vi "Actor Core.vi"(8 "error in":errorcluster, 11 "MonSys_Client_Actor in":refnum<class "MonSys_Client_Actor.lvclass">) -> (0 "error out":errorcluster, 3 "Actor out":refnum<class "Actor.lvclass">)   [LabVIEW 2018, in "MonSys_Client_Actor.lvlib" / "MonSys_Client_Actor.lvclass"]
doc: "(<B>Filename</B>: Actor Framework.lvlib:Actor.lvclass:Actor Core.vi)\n\nReceives messages to the actor, reacts to them, and initiates any error handling that may shut the actor down.\n\nDescendant classes may override this VI to append parallel tasks for the actor to complete while it handles messages. Overrides use the Call Parent Method node."
uses:
  MonSys_Client_Actor.lvclass
  C:/Program Files (x86)/National Instruments/LabVIEW 2018/vi.lib/ActorFramework/Actor/Actor.lvclass
  <vilib>/ActorFramework/Actor/Actor.lvclass
  _MonSys_LIB/OnlineData.ctl
  _MonSys_LIB/OnlineData_State.ctl
  MonSys_Client_Actor.lvclass/MonSys_Client_Actor.ctl
  <vilib>/ActorFramework/Actor/Actor.lvclass/Actor.ctl
  <vilib>/ActorFramework/Message Enqueuer/Message Enqueuer.lvclass/Message Enqueuer.ctl
  <extravilib>/ChannelInstances/Tag-bool/Read With Abort.vi
  <vilib>/ActorFramework/Message Enqueuer/Init from Existing Queue.vi
  <vilib>/ActorFramework/Message Enqueuer/Enqueue.vi
  <extravilib>/ChannelInstances/Tag-bool/Write With Abort.vi
  <vilib>/ActorFramework/Stop Msg/Stop Msg.lvclass
  C:/Program Files (x86)/National Instruments/LabVIEW 2018/vi.lib/ActorFramework/Message/Message.lvclass
  <extravilib>/ChannelInstances/Tag-bool/Instantiate.vi
  <extravilib>/ChannelInstances/Tag-bool/EndpointRead.vi
  <vilib>/ActorFramework/Message Priority Queue/Priority Enqueue.vi
  <extravilib>/ChannelInstances/Tag-bool/Endpoint.vi
  <vilib>/ActorFramework/Message Enqueuer/Message Enqueuer.lvclass
  <vilib>/httpClient/LabVIEWHTTPClient.lvlib
  <extravilib>/ChannelInstances/Tag-bool.lvlib
  _MonSys_LIB/_MonSys_LIB.lvlib
panel:
  out "selected port":string
  out "selected ip address":string
  in  "request_cycle [ms]":u32=1000
  out "web server connection status":string
  out "value":T1 {"OnlineData_State" items=["Idle", "Manually", "Automatic"]}
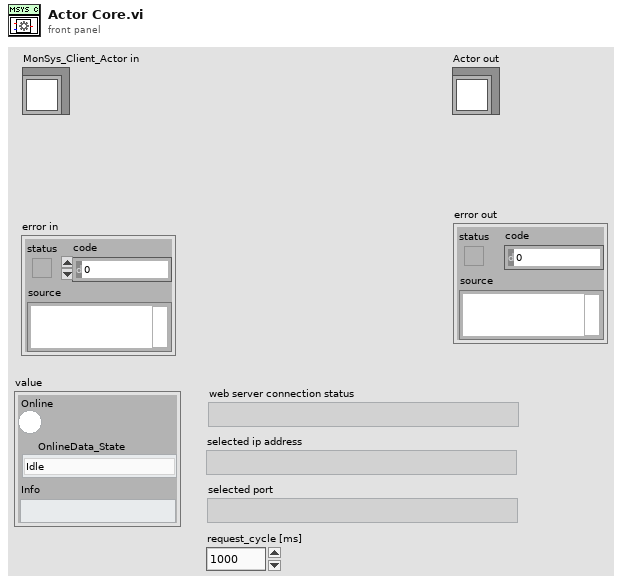
[diagram p1: front panel]
types:
  T1 = typedef "_MonSys_LIB.lvlib/OnlineData.ctl" = cluster{"Online":bool, "Info":string, "OnlineData_State":T2}
  T2 = typedef "_MonSys_LIB.lvlib/OnlineData_State.ctl" = u16
  T3 = enum32{"Invalid", "Standard", "Closed", "Hidden", "Minimized", "Maximized"}
  T4 = typedef "LabVIEWHTTPClient.lvlib/ClientHandle.ctl" = refnum<k1>
  T5 = typedef "Tag-bool.lvlib/))Channel.ctl" = refnum<queue>
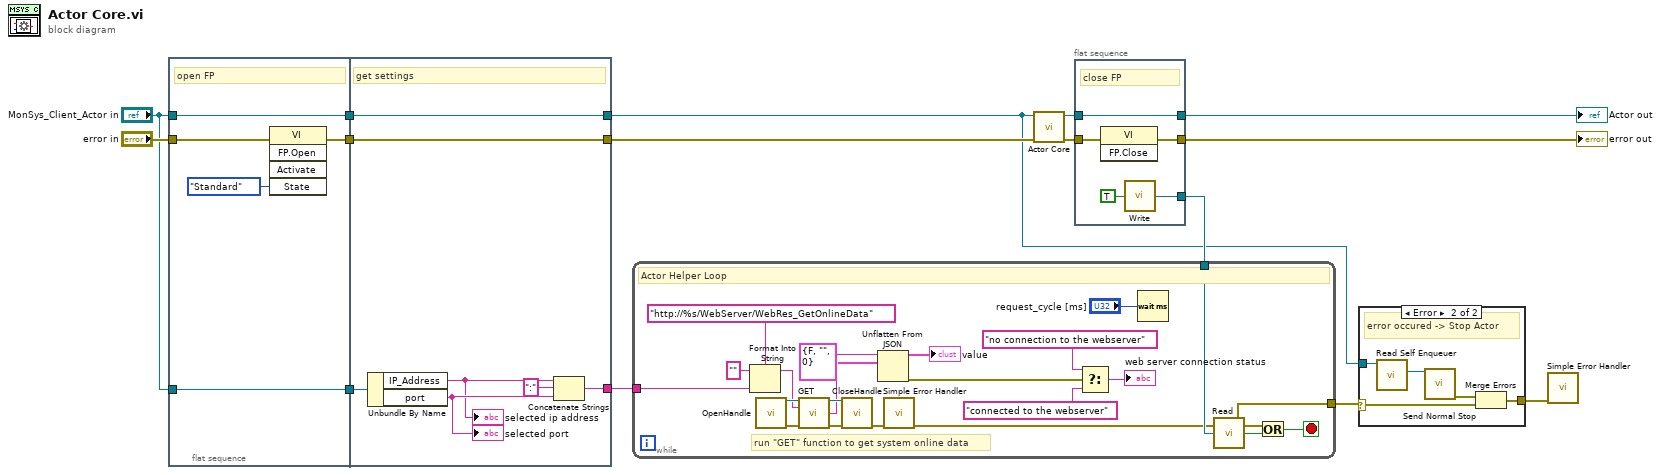
[diagram p0: block diagram]
diagram:
  n1 = flat-sequence {
    tunnel: "MonSys_Client_Actor in" -> [w19]
    tunnel: "MonSys_Client_Actor in" -> [w20]
    tunnel: "error in" -> [w17]
    tunnel: [w16] -> w4
    tunnel: [w20] -> w3
    tunnel: [w19] -> w2
    tunnel: [w21] -> w14
    tunnel: [w27] -> w1
    tunnel: [w22] -> w5
    tunnel: w4 -> [w21]
    tunnel: w3 -> [w27]
    tunnel: w2 -> [w23]
    frame #0 {
      # "open FP"
      n2 = invoke class="VI" method="FP.Open"(error in=w17, "State"=T3."Standard") -> (error out=w16:errorcluster)  [unwired: 3 in, 4 out]
    }
    frame #1 {
      # "get settings"
      n3 = Unbundle By Name(w23) -> ("IP_Address"=w25:string, "port"=w26:string)
      "selected ip address" <- w25
      "selected port" <- w26
      n4 = Concatenate Strings(w25, ":" ("string"), w26) -> (w22:string)
    }
  }
  n5 = while {
    tunnel: w10 -> [w34]
    tunnel: [w32] -> w9
    tunnel: w5 -> [w29]
    stop <- w41 stop-if-true
    # "run \"GET\" function to get system online data"
    # "Actor Helper Loop"
    n6 = Format Into String(format string="http://%s/WebServer/WebRes_GetOnlineData" ("url"), initial string="", w29) -> (resulting string=w28:string)  [unwired: 1 in, 1 out]
    n7 = call <vilib>:"OpenHandle.vi"() -> ("client handle out"=w43:T4, "error out"=w42:errorcluster)  [unwired: 14 in]
    n8 = call <vilib>:"GET.vi"("client handle"=w43, "url"=w28, "error in (no error)"=w42) -> ("client handle out"=w46:T4, "body"=w45:string, "error out"=w32:errorcluster)  [unwired: 9 in, 1 out]
    n9 = call <vilib>:"CloseHandle.vi"("client handle"=w46, "error in (no error)"=w32) -> ("error out"=w47:errorcluster)  [unwired: 13 in]
    n10 = Unflatten From JSON(JSON string=w45, type and defaults=T1 {"Online"=FALSE, "Info"="", "OnlineData_State"=0} ("Data")) -> (value=→"value":T1, error out=w38:errorcluster)  [unwired: 5 in]
    n11 = call <vilib>:"Simple Error Handler.vi"("error in (no error)"=w47) -> ()  [unwired: 4 in, 5 out]
    n12 = Select(t="no connection to the webserver", s=w38, f="connected to the webserver") -> (s? t:f=→"web server connection status":string)
    n13 = Wait (ms)(milliseconds to wait="request_cycle [ms]") -> ()  [unwired: 1 out]
    n14 = call <extravilib>:"Read.vi"("channel"=w34) -> ("element"=w33:bool)  [unwired: 1 in, 1 out]
    n15 = Or(x=w32, y=w33) -> (x .or. y?=w41:bool)
  }
  n16 = call-parent "Actor Core.vi"("error in"=w14, "Actor in"=w1) -> ("error out"=w12:errorcluster, "Actor out"=w13:refnum<class "Actor.lvclass">)  [unwired: 8 in]
  n17 = flat-sequence {
    tunnel: [w52] -> w7
    tunnel: w13 -> [w52]
    tunnel: w12 -> [w51]
    tunnel: [w50] -> w11
    tunnel: [w48] -> w10
    frame #0 {
      # "close FP"
      n18 = invoke class="VI" method="FP.Close"(error in=w51) -> (error out=w50:errorcluster)  [unwired: 2 in, 2 out]
      n19 = call <extravilib>:"Write.vi"("element"=TRUE) -> ("channel"=w48:T5)  [unwired: 1 out]
    }
  }
  n20 = case shown="Error" w9 {
    selector: w9 -> [w53 w57]
    tunnel: [w53 w56] -> w8
    tunnel: w1 -> [_ w55]
    frame No Error {
    }
    frame Error {
      # "error occured -> Stop Actor"
      n21 = call <vilib>:"Read Self Enqueuer.vi"("Actor"=w55) -> ("Self Enqueuer"=w54:refnum<class "Message Enqueuer.lvclass">)  [unwired: 10 in]
      n22 = call <vilib>:"Send Normal Stop.vi"("Message Enqueuer"=w54) -> ("error out"=w58:errorcluster)  [unwired: 10 in]
      n23 = Merge Errors(w58, w57) -> (w56:errorcluster)
    }
  }
  n24 = call <vilib>:"Simple Error Handler.vi"("error in (no error)"=w8) -> ()  [unwired: 4 in, 5 out]
  "error out" <- w11
  "Actor out" <- w7
